vi "Fix Relocated Modules.vi"(8 "error in (no error)":errorcluster, 11 "Routing and Faulting Ref in":T1 format="%.0x") -> (0 "error out":errorcluster, 3 "Routing and Faulting Ref out":T1 format="%.0x")   [LabVIEW 2017, in "Routing and Faulting Scripting.lvlib"]
uses:
  Routing and Faulting Scripting.lvlib
  <vilib>/NI Veristand/Custom Device API/Custom Device Item Ref.ctl
  <vilib>/NI Veristand/Custom Device API/Custom Device API.lvlib
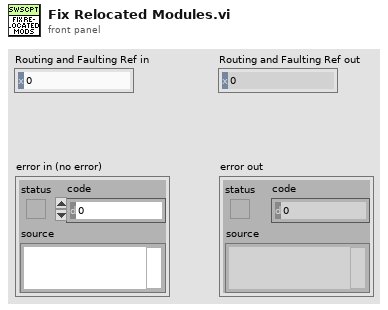
[diagram p1: front panel]
types:
  T1 = typedef "Custom Device API.lvlib/Custom Device Item Ref.ctl" = u64
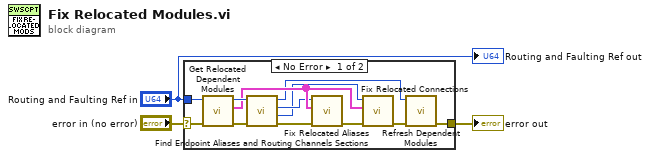
[diagram p0: block diagram]
diagram:
  n1 = case shown="No Error" "error in (no error)" {
    selector: "error in (no error)" -> [w10 w16]
    tunnel: "Routing and Faulting Ref in" -> [w12 _]
    tunnel: [w11 w16] -> w3
    frame No Error {
      n2 = call "Get Relocated Dependent Modules.vi"("error in (no error)"=w10, "Routing and Faulting Ref in"=w12) -> ("error out"=w15:errorcluster, "Outdated Dependent Modules"=w7:cluster{"Old Path":string, "New Path":string}[], "Routing and Faulting Ref out"=w14:T1)  [unwired: 6 in, 1 out]
      n3 = call "Find Endpoint Aliases and Routing Channels Sections.vi"("error in (no error)"=w15, "Routing and Faulting Custom Device Ref in"=w14) -> ("error out"=w8:errorcluster, "Routing Channels Ref"=w5:T1, "Endpoint Aliases Ref"=w6:T1, "Routing and Faulting Custom Device Ref out"=w4:T1)  [unwired: 6 in]
      n4 = call "Fix Relocated Aliases.vi"("error in (no error)"=w8, "Outdated Dependent Modules"=w7, "Endpoint Aliases Ref in"=w6) -> ("error out"=w9:errorcluster)  [unwired: 7 in, 1 out]
      n5 = call "Fix Relocated Connections.vi"("error in (no error)"=w9, "Outdated Dependent Modules"=w7, "Routing Channels Ref in"=w5) -> ("error out"=w13:errorcluster)  [unwired: 7 in, 1 out]
      n6 = call "Refresh Dependent Modules.vi"("error in (no error)"=w13, "Routing and Faulting Ref in"=w4) -> ("error out"=w11:errorcluster)  [unwired: 8 in, 1 out]
    }
    frame Error {
    }
  }
  "error out" <- w3
  "Routing and Faulting Ref out" <- "Routing and Faulting Ref in"
